vi "BMM LIN Init.vi"(9 "BaudRate":i32, 10 "LINIndex":u8, 11 "DevHandle":i32) -> (3 "function return":i32)   [LabVIEW 2010, in "usb2bmm_lin.lvlib"]
doc: "int WINAPI BMM_LIN_Init(int DevHandle,unsigned char LINIndex,int BaudRate);"
uses:
  usb2bmm_lin.lvlib
  USB2XXX/trunk/USB2XXX/USB2XXX/vs2019/Release/USB2XXX.dll
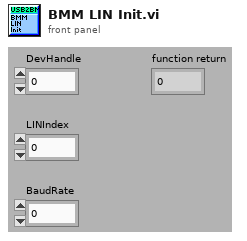
[diagram p1: front panel]
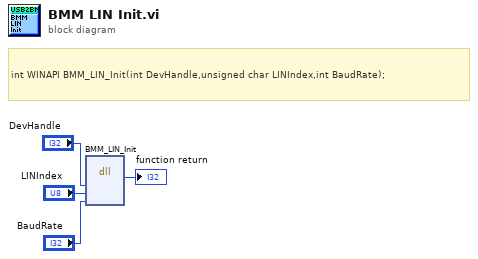
[diagram p0: block diagram]
diagram:
  # "int WINAPI BMM_LIN_Init(int DevHandle,unsigned char LINIndex,int BaudRate);"
  n1 = dll-call lib="E:/Projects/USB2XXX/trunk/USB2XXX/USB2XXX/vs2019/Release/USB2XXX.*" fn="BMM_LIN_Init"("DevHandle"="DevHandle", "LINIndex"="LINIndex", "BaudRate"="BaudRate") -> (→"function return":i32)  [unwired: 6 in, 2 out]
